vi "Error Handler - DTACQ Mid Level.vi"(8 "error in":errorcluster, 11 "DTACQ Connection Data In":T1={"Description"="", "Address"="", "Port"=0, "timeout (ms)"=5000, "Termination Character"="\n", "TCP Connection Reference"=refnum, "Open Connection"=FALSE}) -> (0 "error out":errorcluster, 2 "Timed Out":bool, 3 "DTACQ Connection Data Out":T1={"Description"="", "Address"="", "Port"=0, "timeout (ms)"=5000, "Termination Character"="\n", "TCP Connection Reference"=refnum, "Open Connection"=FALSE})   [LabVIEW 2017, in "Communications Library.lvlib"]
doc: "Error handler for the DTACQ driver. \n\nAny unhandled error will remain, after running this VI. Handled errors will be downgraded to a warning.\n\nHandles the following errors;\n56 - TCP Timeout error\n66 - Unexpected close of TCP connection\n5101 - Unexpected response"
uses:
  Communications Library.lvlib
  Typedefs/DTACQ Connection Data--Cluster.ctl
  Debug - Lower Level - Logging Tool.vi
  Error 5102 - DTACQ unit replied with an error--const.vi
  <vilib>/Utility/error.llb/Error Cluster From Error Code.vi
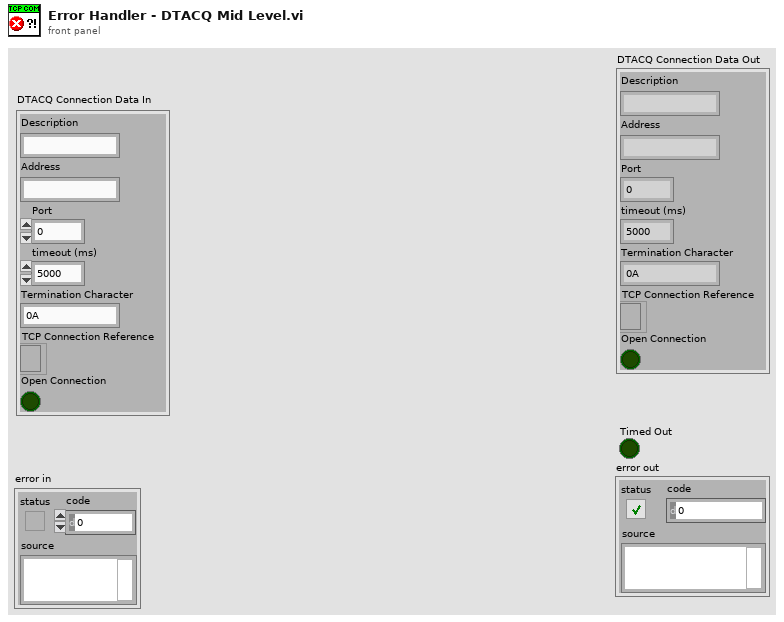
[diagram p1: front panel]
types:
  T1 = typedef "Communications Library.lvlib/DTACQ Connection Data--Cluster.ctl" = cluster{"Description":string, "Address":string, "Port":u16, "timeout (ms)":i32, "Termination Character":string, "TCP Connection Reference":refnum<k5>, "Open Connection":bool}
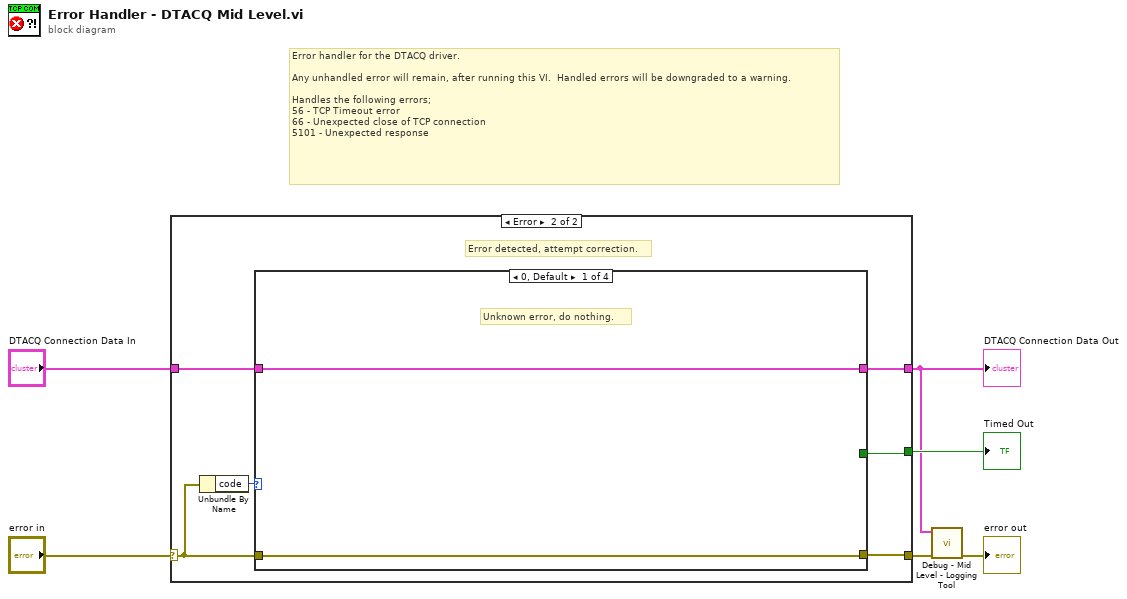
[diagram p0: block diagram]
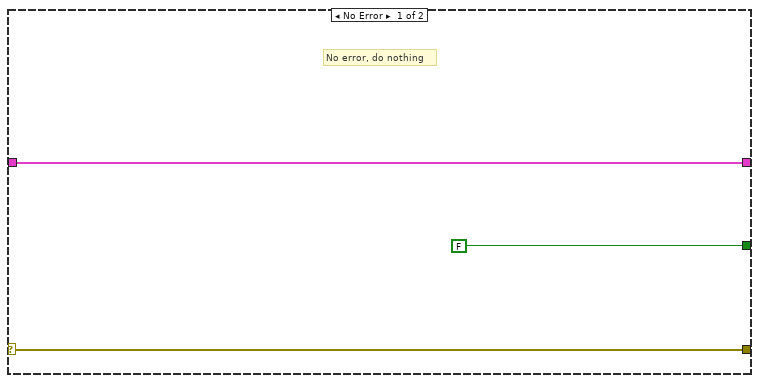
[diagram p2: hidden frame]
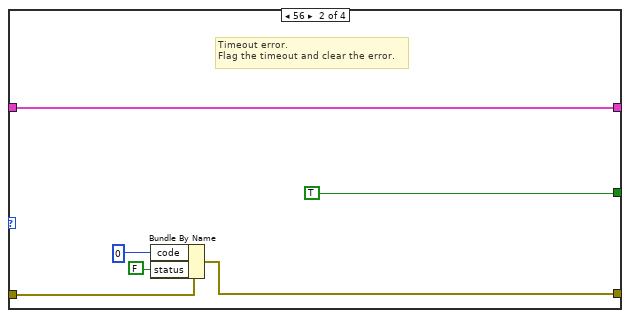
[diagram p3: hidden frame]
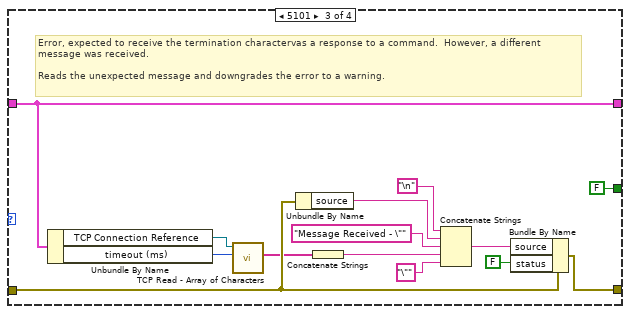
[diagram p4: hidden frame]
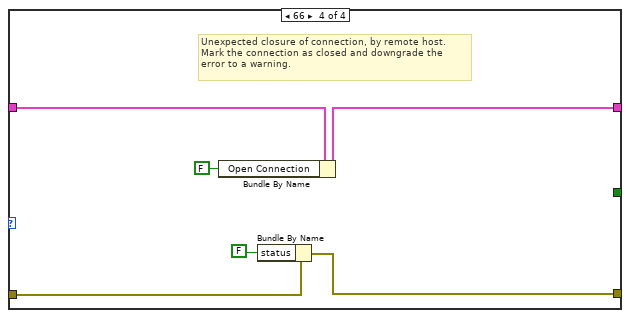
[diagram p5: hidden frame]
diagram:
  # "Error handler for the DTACQ driver.  \n\nAny unhandled error will remain, after running this VI.  Handled errors will be downgraded to a warning.\n\nHandles the following errors;\n56 - TCP Timeout error\n66 - Unexpected close of TCP connection\n5101 - Unexpected response"
  n1 = case shown="Error" "error in" {
    selector: "error in" -> [w8 w13]
    tunnel: "DTACQ Connection Data In" -> [w9 w15]
    tunnel: [w9 w11] -> w1
    tunnel: [w8 w12] -> w3
    tunnel: [FALSE w10] -> w5
    frame No Error {
      # "No error, do nothing"
    }
    frame Error {
      # "Error detected, attempt correction."
      n2 = Unbundle By Name(w13) -> ("code"=w14:i32)
      n3 = case shown="0, Default" w14 {
        tunnel: w15 -> [w16 w23 w36 w40]
        tunnel: w13 -> [w17 w20 w32 w43]
        tunnel: [w17 w19 w31 w41] -> w12
        tunnel: [w16 w23 w36 w38] -> w11
        tunnel: [_ TRUE FALSE _] -> w10
        frame 0, Default {
          # "Unknown error, do nothing."
        }
        frame 56 {
          # "Timeout error.\nFlag the timeout and clear the error."
          n4 = Bundle By Name(cluster=w20, "code"=0, "status"=FALSE) -> (w19:errorcluster)
        }
        frame 5101 {
          # "Error, expected to receive the termination charactervas a response to a command.  However, a different\nmessage was received.  \n\nReads the unexpected message and downgrades the error to a warning."
          n5 = Unbundle By Name(w36) -> ("TCP Connection Reference"=w28:refnum<k5>, "timeout (ms)"=w27:i32)
          n6 = call "TCP Read - Array of Characters.vi"("timeout ms (default 50ms)"=w27, "TCP Network Connection in"=w28) -> ("Characters Read"=w26:string[])  [unwired: 7 in, 2 out]
          n7 = Unbundle By Name(w32) -> ("source"=w33:string)
          n8 = Concatenate Strings(w26) -> (w25:string)
          n9 = Concatenate Strings("\n", w33, "Message Received - \"", w25, "\"") -> (w30:string)
          n10 = Bundle By Name(cluster=w32, "source"=w30, "status"=FALSE) -> (w31:errorcluster)
        }
        frame 66 {
          # "Unexpected closure of connection, by remote host.\nMark the connection as closed and downgrade the\nerror to a warning."
          n11 = Bundle By Name(cluster=w40, "Open Connection"=FALSE) -> (w38:T1)
          n12 = Bundle By Name(cluster=w43, "status"=FALSE) -> (w41:errorcluster)
        }
      }
    }
  }
  "DTACQ Connection Data Out" <- w1
  "Timed Out" <- w5
  n13 = call "Debug - Mid Level - Logging Tool.vi"("Error In"=w3, "DTACQ Connection Data In"=w1) -> ("Error Out"=→"error out":errorcluster)  [unwired: 8 in, 1 out]
